vi "dcamrecord_MM.vi"(7 "IntensityGraph in":refnum<vi>, 8 "error in (no error)":errorcluster {"code" format="%.0x"}, 10 "Frames number":i32=10, 11 "Handle in":u32) -> (0 "error out":errorcluster {"code" format="%.0x"}, 1 "subarray":u16[][](graph), 3 "Handle out":u32)   [LabVIEW 2015]
panel:
  out "Frame index":i32
  out "Frame Count":i32
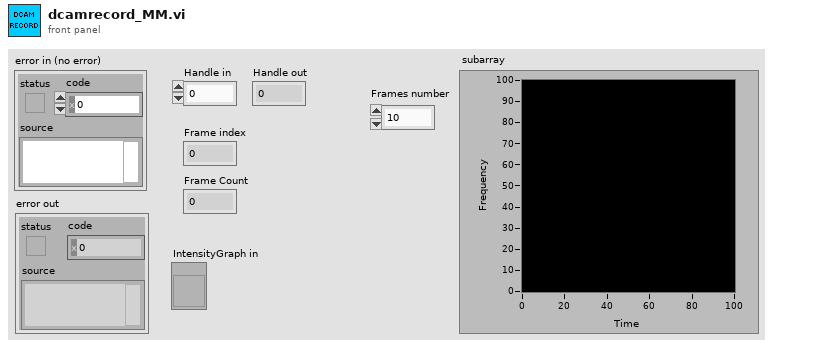
[diagram p1: front panel]
types:
  T1 = cluster{"height":u32, "width":u32, "datatype":u32}
  T2 = cluster{"Value":i32, "Minimum":i32, "Maximum":i32, "Increment":i32}
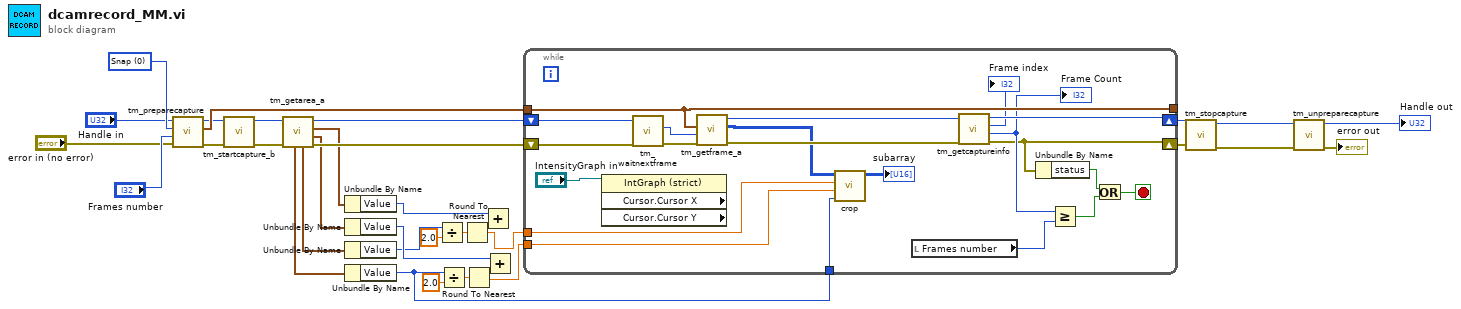
[diagram p0: block diagram]
diagram:
  w25 = 0 items=["Snap", "Sequence"] ("Capture mode")
  n1 = call <userlib>:"tm_preparecapture.vi"("error in (no error)"="error in (no error)", "Frames"="Frames number", "Capture mode"=w25, "Handle in"="Handle in") -> ("error out"=w27:errorcluster, "Buffer Info"=w28:T1, "Handle out"=w26:u32)  [unwired: 4 in, 1 out]
  n2 = call <userlib>:"tm_startcapture_b.vi"("error in (no error)"=w27, "Handle in"=w26) -> ("error out"=w11:errorcluster, "Handle out"=w13:u32)  [unwired: 8 in]
  n3 = call <userlib>:"tm_getarea_a.vi"("error in (no error)"=w11, "Handle in"=w13) -> ("error out"=w10:errorcluster, "V Offset"=w8:T2, "H Offset"=w9:T2, "Handle out"=w12:u32, "H Width"=w7:T2, "V Width"=w6:T2)  [unwired: 4 in]
  n4 = Unbundle By Name(w9) -> ("Value"=w17:i32)
  n5 = Unbundle By Name(w8) -> ("Value"=w14:i32)
  n6 = Unbundle By Name(w7) -> ("Value"=w5:i32)
  n7 = Unbundle By Name(w6) -> ("Value"=w1:i32)
  n8 = Divide(x=w5, y=2.0) -> (x/y=w3:dbl)
  n9 = Divide(x=w1, y=2.0) -> (x/y=w16:dbl)
  n10 = Round To Nearest(number=w3) -> (nearest integer value=w2:dbl)
  n11 = Round To Nearest(number=w16) -> (nearest integer value=w4:dbl)
  n12 = Add(x=w17, y=w2) -> ()  [unwired: 1 out]
  n13 = Add(x=w14, y=w4) -> ()  [unwired: 1 out]
  n14 = while {
    tunnel: w28 -> [w45]
    tunnel: [w45] -> _
    shift-right: [w47] -> w24
    shift-left: w12 -> [w52]
    shift-right: [w37] -> w23
    shift-left: w10 -> [w51]
    tunnel: w2 -> [w34]
    tunnel: w4 -> [w33]
    tunnel: w1 -> [w32]
    stop <- w48 stop-if-true
    n15 = property class="IntGraph (strict)" props=["Cursor", "Cursor X", "Cursor", "Cursor Y"](reference="IntensityGraph in") -> ()  [unwired: 1 in, 4 out]
    n16 = call <userlib>:"tm_waitnextframe.vi"("error in (no error)"=w51, "Handle in"=w52) -> ("error out"=w49:errorcluster, "Frame Index"=w42:i32)  [unwired: 6 in, 2 out]
    n17 = call <userlib>:"tm_getframe_a.vi"("error in (no error)"=w49, "Frame Index"=w42, "Buffer Info"=w45) -> ("error out"=w46:errorcluster, "Data 16"=w40:u16[][], "Handle out"=w50:u32)  [unwired: 4 in, 2 out]
    n18 = call "crop.vi"("boxsize"=w32, "Y"=w33, "X"=w34, "Data 16"=w40) -> ("Array"=→"subarray":u16[][])  [unwired: 7 in]
    n19 = local read "Frames number"() -> (w41:i32)
    n20 = call <userlib>:"tm_getcaptureinfo.vi"("error in (no error)"=w46, "Handle in"=w50) -> ("error out"=w37:errorcluster, "Frame Count"=w43:i32, "Frame Index"=→"Frame index":i32, "Handle out"=w47:u32)  [unwired: 6 in]
    "Frame Count" <- w43
    n21 = Unbundle By Name(w37) -> ("status"=w36:bool)
    n22 = Greater Or Equal?(x=w43, y=w41) -> (x >= y?=w38:bool)
    n23 = Or(x=w36, y=w38) -> (x .or. y?=w48:bool)
  }
  n24 = call <userlib>:"tm_stopcapture.vi"("error in (no error)"=w23, "Handle in"=w24) -> ("error out"=w30:errorcluster, "Handle out"=w31:u32)  [unwired: 8 in]
  n25 = call <userlib>:"tm_unpreparecapture.vi"("error in (no error)"=w30, "Handle in"=w31) -> ("error out"=→"error out":errorcluster, "Handle out"=→"Handle out":u32)  [unwired: 8 in]
